vi "read default menu name.vi"(8 "error in":errorcluster, 11 "Shared Library Module editor node in":refnum<class "Shared Library Module editor node.lvclass">) -> (0 "error out":errorcluster, 2 "default menu name":string, 3 "Shared Library Module editor node out":refnum<class "Shared Library Module editor node.lvclass">)   [LabVIEW 2013, in "Shared Library Module editor node.lvclass"]
uses:
  Shared Library Module editor node.lvclass
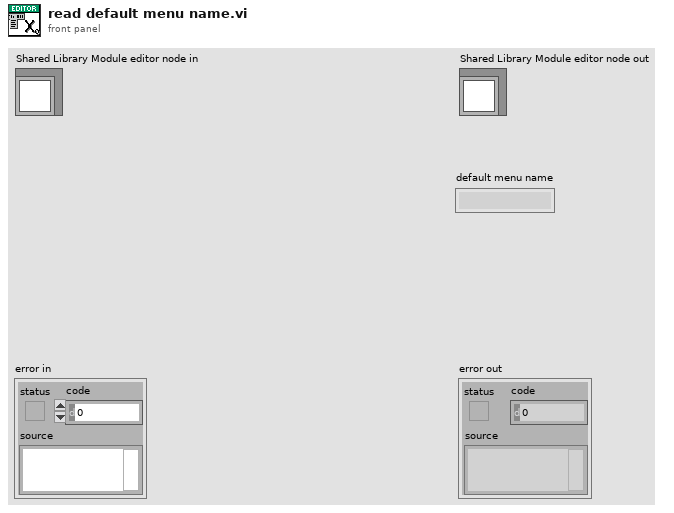
[diagram p1: front panel]
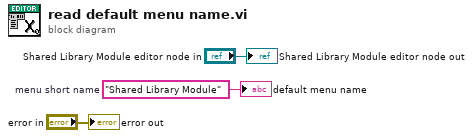
[diagram p0: block diagram]
diagram:
  w3 = "Shared Library Module"  # menu short name
  "error out" <- "error in"
  "Shared Library Module editor node out" <- "Shared Library Module editor node in"
  "default menu name" <- w3
